vi "rsscope_core_global.vi"() -> ()   [LabVIEW 2014] (continued)
"Flags"=0, "Help"="DefiDefines, whether a search for any word length error (too few or too many bits per word) shall be activated or not.\n\nAvailable Repeated Capabilities:\nNone\n\nRemote-control command(s):\nSEARch:TRIGger:ETHernet:ERRor:LENGth"}, {"Level"=4, "Class Only"=TRUE, "Identifier"="", "Descriptive Name"="Results", "Data Type"=0, "Command"="", "Access"=0, "Range Table"="", "Read Callback"="", "Write Callback"="", "Supported Models"="", "Instrument Options"="", "Flags"=0, "Help"="Returns the search result of the specified word."}, {"Level"=5, "Class Only"=FALSE, "Identifier"="RSSCOPE_ATTR_SEARCH_ETHERNET_WORD_COUNT", "Descriptive Name"="Search Ethernet Word Count", "Data Type"=0, "Command"="SEAR:RES:ETH:WCO?", "Access"=0, "Range Table"="", "Read Callback"="rsscope_FormatSearchNameInt32_ReadCallback.vi", "Write Callback"="", "Supported Models"="", "Instrument Options"="K8", "Flags"=0, "Help"="Returns the number of decoded words.\n\nAvailable Repeated Capabilities:\nNone\n\nRemote-control command(s):\nSEARch:RESult:ETHernet:WCOunt?"}, {"Level"=3, "Class Only"=TRUE, "Identifier"="", "Descriptive Name"="USB", "Data Type"=0, "Command"="", "Access"=0, "Range Table"="", "Read Callback"="", "Write Callback"="", "Supported Models"="", "Instrument Options"="", "Flags"=0, "Help"="Configures USB search settings."}, {"Level"=4, "Class Only"=FALSE, "Identifier"="RSSCOPE_ATTR_SEARCH_USB_CRITERIA_START_OF_PACKET", "Descriptive Name"="Search USB Criteria Start Of Packet", "Data Type"=3, "Command"="SEAR:TRIG:USB:SSOP", "Access"=2, "Range Table"="", "Read Callback"="rsscope_FormatSearchNameBoolean_ReadCallback.vi", "Write Callback"="rsscope_FormatSearchNameBoolean_WriteCallback.vi", "Supported Models"="", "Instrument Options"="K60", "Flags"=0, "Help"="Defines, whether a start of packet (SOP) search shall be activated or not.\n\nAvailable Repeated Capabilities:\nNone\n\nRemote-control command(s):\nSEARch:TRIGger:USB:SSOP"}, {"Level"=4, "Class Only"=FALSE, "Identifier"="RSSCOPE_ATTR_SEARCH_USB_CRITERIA_TOKEN", "Descriptive Name"="Search USB Criteria Token", "Data Type"=3, "Command"="SEAR:TRIG:USB:STOK", "Access"=2, "Range Table"="", "Read Callback"="rsscope_FormatSearchNameBoolean_ReadCallback.vi", "Write Callback"="rsscope_FormatSearchNameBoolean_WriteCallback.vi", "Supported Models"="", "Instrument Options"="K60", "Flags"=0, "Help"="Defines, whether a search for any token packet shall be activated or not.\n\nAvailable Repeated Capabilities:\nNone\n\nRemote-control command(s):\nSEARch:TRIGger:USB:STOKen"}, {"Level"=4, "Class Only"=FALSE, "Identifier"="RSSCOPE_ATTR_SEARCH_USB_CRITERIA_DATA", "Descriptive Name"="Search USB Criteria Data", "Data Type"=3, "Command"="SEAR:TRIG:USB:SDAT", "Access"=2, "Range Table"="", "Read Callback"="rsscope_FormatSearchNameBoolean_ReadCallback.vi", "Write Callback"="rsscope_FormatSearchNameBoolean_WriteCallback.vi", "Supported Models"="", "Instrument Options"="K60", "Flags"=0, "Help"="Defines, whether the search for any data packet shall be activated or not.\n\nAvailable Repeated Capabilities:\nNone\n\nRemote-control command(s):\nSEARch:TRIGger:USB:SDATa"}, {"Level"=4, "Class Only"=FALSE, "Identifier"="RSSCOPE_ATTR_SEARCH_USB_CRITERIA_HANDSHAKE", "Descriptive Name"="Search USB Criteria Handshake", "Data Type"=3, "Command"="SEAR:TRIG:USB:SHAN", "Access"=2, "Range Table"="", "Read Callback"="rsscope_FormatSearchNameBoolean_ReadCallback.vi", "Write Callback"="rsscope_FormatSearchNameBoolean_WriteCallback.vi", "Supported Models"="", "Instrument Options"="K60", "Flags"=0, "Help"="Defines, whether the search for any handshake packet shall be activated or not.\n\nAvailable Repeated Capabilities:\nNone\n\nRemote-control command(s):\nSEARch:TRIGger:USB:SHANdshake"}, {"Level"=4, "Class Only"=FALSE, "Identifier"="RSSCOPE_ATTR_SEARCH_USB_CRITERIA_SPECIAL_PID", "Descriptive Name"="Search USB Criteria Special PID", "Data Type"=3, "Command"="SEAR:TRIG:USB:SSPE", "Access"=2, "Range Table"="", "Read Callback"="rsscope_FormatSearchNameBoolean_ReadCallback.vi", "Write Callback"="rsscope_FormatSearchNameBoolean_WriteCallback.vi", "Supported Models"="", "Instrument Options"="K60", "Flags"=0, "Help"="Defines, whether the search for any special PID packet shall be activated or not.\n\nAvailable Repeated Capabilities:\nNone\n\nRemote-control command(s):\nSEARch:TRIGger:USB:SSPE"}, {"Level"=4, "Class Only"=FALSE, "Identifier"="RSSCOPE_ATTR_SEARCH_USB_CRITERIA_ERROR", "Descriptive Name"="Search USB Criteria Error", "Data Type"=3, "Command"="SEAR:TRIG:USB:SERR", "Access"=2, "Range Table"="", "Read Callback"="rsscope_FormatSearchNameBoolean_ReadCallback.vi", "Write Callback"="rsscope_FormatSearchNameBoolean_WriteCallback.vi", "Supported Models"="", "Instrument Options"="K60", "Flags"=0, "Help"="Defines, whether the search for any error condition shall be activated or not.\n\nAvailable Repeated Capabilities:\nNone\n\nRemote-control command(s):\nSEARch:TRIGger:USB:SERRor"}, {"Level"=4, "Class Only"=FALSE, "Identifier"="RSSCOPE_ATTR_SEARCH_USB_TOKEN", "Descriptive Name"="Search USB Token", "Data Type"=0, "Command"="SEAR:TRIG:USB:TOK", "Access"=2, "Range Table"="rsscope_rngProtocolUSBSearchToken", "Read Callback"="rsscope_FormatSearchNameInt32_ReadCallback.vi", "Write Callback"="rsscope_FormatSearchNameInt32_WriteCallback.vi", "Supported Models"="", "Instrument Options"="K60", "Flags"=0, "Help"="Defines which token packet type is searched for: Out, In, Start Of Frame, Setup, or any token packet.\n\nAvailable Repeated Capabilities:\nNone\n\nRemote-control command(s):\nSEARch:TRIGger:USB:TOKen"}, {"Level"=4, "Class Only"=FALSE, "Identifier"="RSSCOPE_ATTR_SEARCH_USB_DATA_TYPE", "Descriptive Name"="Search USB Data Type", "Data Type"=0, "Command"="SEAR:TRIG:USB:DATA", "Access"=2, "Range Table"="rsscope_rngProtocolUSBSearchDataType", "Read Callback"="rsscope_FormatSearchNameInt32_ReadCallback.vi", "Write Callback"="rsscope_FormatSearchNameInt32_WriteCallback.vi", "Supported Models"="", "Instrument Options"="K60", "Flags"=0, "Help"="Defines, which data packet type is searched for: &apos;DATA0&apos;, &apos;DATA1&apos;, &apos;DATA2&apos;, or &apos;MDATA&apos;, as well as &apos;Any&apos; data packet.\n\nAvailable Repeated Capabilities:\nNone\n\nRemote-control command(s):\nSEARch:TRIGger:USB:DATA"}, {"Level"=4, "Class Only"=FALSE, "Identifier"="RSSCOPE_ATTR_SEARCH_USB_HANDSHAKE", "Descriptive Name"="Search USB Handshake", "Data Type"=0, "Command"="SEAR:TRIG:USB:HAND", "Access"=2, "Range Table"="rsscope_rngProtocolUSBTriggerHandshake", "Read Callback"="rsscope_FormatSearchNameInt32_ReadCallback.vi", "Write Callback"="rsscope_FormatSearchNameInt32_WriteCallback.vi", "Supported Models"="", "Instrument Options"="", "Flags"=0, "Help"="Defines, which handshake type is searched for.\n\nAvailable Repeated Capabilities:\nNone\n\nRemote-control command(s):\nSEARch:TRIGger:USB:HAND"}, {"Level"=4, "Class Only"=FALSE, "Identifier"="RSSCOPE_ATTR_SEARCH_USB_SPECIAL_PID", "Descriptive Name"="Search USB Special PID", "Data Type"=0, "Command"="SEAR:TRIG:USB:SPEC", "Access"=2, "Range Table"="rsscope_rngProtocolUSBSearchSpecialPID", "Read Callback"="rsscope_FormatSearchNameInt32_ReadCallback.vi", "Write Callback"="rsscope_FormatSearchNameInt32_WriteCallback.vi", "Supported Models"="", "Instrument Options"="K60", "Flags"=0, "Help"="Defines, which special PID packet type is searched for: &apos;PREamble&apos;, &apos;ERR&apos;, &apos;SPLit&apos;, &apos;PING&apos;, or &apos;Any&apos; special PID packet.\n\nAvailable Repeated Capabilities:\nNone\n\nRemote-control command(s):\nSEARch:TRIGger:USB:SPEC"}, {"Level"=4, "Class Only"=FALSE, "Identifier"="RSSCOPE_ATTR_SEARCH_USB_PID_ERROR_CHECK", "Descriptive Name"="Search USB PID Error Check", "Data Type"=3, "Command"="SEAR:TRIG:USB:WPID", "Access"=2, "Range Table"="", "Read Callback"="rsscope_FormatSearchNameBoolean_ReadCallback.vi", "Write Callback"="rsscope_FormatSearchNameBoolean_WriteCallback.vi", "Supported Models"="", "Instrument Options"="K60", "Flags"=0, "Help"="Defines, whether the packet ID error check shall be activated or not.\n\nAvailable Repeated Capabilities:\nNone\n\nRemote-control command(s):\nSEARch:TRIGger:USB:WPID"}, {"Level"=4, "Class Only"=TRUE, "Identifier"="", "Descriptive Name"="Error Condition", "Data Type"=0, "Command"="", "Access"=0, "Range Table"="", "Read Callback"="", "Write Callback"="", "Supported Models"="", "Instrument Options"="", "Flags"=0, "Help"="Configures error conditions to be searched."}, {"Level"=5, "Class Only"=FALSE, "Identifier"="RSSCOPE_ATTR_SEARCH_USB_ERROR_PID", "Descriptive Name"="Search USB Error PID", "Data Type"=3, "Command"="SEAR:TRIG:USB:PID", "Access"=2, "Range Table"="", "Read Callback"="rsscope_FormatSearchNameBoolean_ReadCallback.vi", "Write Callback"="rsscope_FormatSearchNameBoolean_WriteCallback.vi", "Supported Models"="", "Instrument Options"="K60", "Flags"=0, "Help"="Defines, whether a search for any PID error shall be activated or not.\n\nAvailable Repeated Capabilities:\nNone\n\nRemote-control command(s):\nSEARch:TRIGger:USB:PIDerror"}, {"Level"=5, "Class Only"=FALSE, "Identifier"="RSSCOPE_ATTR_SEARCH_USB_ERROR_CRC5", "Descriptive Name"="Search USB Error CRC5", "Data Type"=3, "Command"="SEAR:TRIG:USB:CRC5error", "Access"=2, "Range Table"="", "Read Callback"="rsscope_FormatSearchNameBoolean_ReadCallback.vi", "Write Callback"="rsscope_FormatSearchNameBoolean_WriteCallback.vi", "Supported Models"="", "Instrument Options"="K60", "Flags"=0, "Help"="Defines, whether a search for any CRC5 error shall be activated or not.\n\nAvailable Repeated Capabilities:\nNone\n\nRemote-control command(s):\nSEARch:TRIGger:USB:CRC5error"}, {"Level"=5, "Class Only"=FALSE, "Identifier"="RSSCOPE_ATTR_SEARCH_USB_ERROR_CRC16", "Descriptive Name"="Search USB Error CRC16", "Data Type"=3, "Command"="SEAR:TRIG:USB:CRC16error", "Access"=2, "Range Table"="", "Read Callback"="rsscope_FormatSearchNameBoolean_ReadCallback.vi", "Write Callback"="rsscope_FormatSearchNameBoolean_WriteCallback.vi", "Supported Models"="", "Instrument Options"="K60", "Flags"=0, "Help"="Defines, whether a search for any CRC16 error shall be activated or not.\n\nAvailable Repeated Capabilities:\nNone\n\nRemote-control command(s):\nSEARch:TRIGger:USB:CRC16error"}, {"Level"=5, "Class Only"=FALSE, "Identifier"="RSSCOPE_ATTR_SEARCH_USB_ERROR_BITSTUFF", "Descriptive Name"="Search USB Error Bitstuff", "Data Type"=3, "Command"="SEAR:TRIG:USB:BITS", "Access"=2, "Range Table"="", "Read Callback"="rsscope_FormatSearchNameBoolean_ReadCallback.vi", "Write Callback"="rsscope_FormatSearchNameBoolean_WriteCallback.vi", "Supported Models"="", "Instrument Options"="K60", "Flags"=0, "Help"="Defines, whether a search for any bitstuffing error shall be activated or not.\n\nAvailable Repeated Capabilities:\nNone\n\nRemote-control command(s):\nSEARch:TRIGger:USB:BITSterror"}, {"Level"=5, "Class Only"=FALSE, "Identifier"="RSSCOPE_ATTR_SEARCH_USB_ERROR_GLITCH", "Descriptive Name"="Search USB Error Glitch", "Data Type"=3, "Command"="SEAR:TRIG:USB:GLIT", "Access"=2, "Range Table"="", "Read Callback"="rsscope_FormatSearchNameBoolean_ReadCallback.vi", "Write Callback"="rsscope_FormatSearchNameBoolean_WriteCallback.vi", "Supported Models"="", "Instrument Options"="K60", "Flags"=0, "Help"="Defines, whether a search for any glitch error shall be activated or not.\n\nAvailable Repeated Capabilities:\nNone\n\nRemote-control command(s):\nSEARch:TRIGger:USB:GLITcherror"}, {"Level"=4, "Class Only"=TRUE, "Identifier"="", "Descriptive Name"="End Point Check", "Data Type"=0, "Command"="", "Access"=0, "Range Table"="", "Read Callback"="", "Write Callback"="", "Supported Models"="", "Instrument Options"="", "Flags"=0, "Help"="Defines, whether an endpoint check that meets specific conditions is executed or not."}, {"Level"=5, "Class Only"=FALSE, "Identifier"="RSSCOPE_ATTR_SEARCH_USB_END_POINT_CHECK", "Descriptive Name"="Search USB End Point Check", "Data Type"=3, "Command"="SEAR:TRIG:USB:WEND", "Access"=2, "Range Table"="", "Read Callback"="rsscope_FormatSearchNameBoolean_ReadCallback.vi", "Write Callback"="rsscope_FormatSearchNameBoolean_WriteCallback.vi", "Supported Models"="", "Instrument Options"="K60", "Flags"=0, "Help"="Defines, whether the endpoint check shall be activated or not.\n\nAvailable Repeated Capabilities:\nNone\n\nRemote-control command(s):\nSEARch:TRIGger:USB:WEND"}, {"Level"=5, "Class Only"=FALSE, "Identifier"="RSSCOPE_ATTR_SEARCH_USB_END_POINT_CHECK_CONDITION", "Descriptive Name"="Search USB End Point Check Condition", "Data Type"=0, "Command"="SEAR:TRIG:USB:ECON", "Access"=2, "Range Table"="rsscope_rngProtocolTriggerCondition", "Read Callback"="rsscope_FormatSearchNameInt32_ReadCallback.vi", "Write Callback"="rsscope_FormatSearchNameInt32_WriteCallback.vi", "Supported Models"="", "Instrument Options"="K60", "Flags"=0, "Help"="Sets the operator to set a specific endpoint or an endpoint range.\n\nAvailable Repeated Capabilities:\nNone\n\nRemote-control command(s):\nSEARch:TRIGger:USB:ECONdition"}, {"Level"=5, "Class Only"=FALSE, "Identifier"="RSSCOPE_ATTR_SEARCH_USB_END_POINT_CHECK_MIN", "Descriptive Name"="Search USB End Point Check Min", "Data Type"=2, "Command"="SEAR:TRIG:USB:EMIN", "Access"=1, "Range Table"="", "Read Callback"="", "Write Callback"="rsscope_FormatSearchNameString_WriteCallback.vi", "Supported Models"="", "Instrument Options"="K60", "Flags"=0, "Help"="Specifies the endpoint, or sets the start value of an endpoint range.\n\nAvailable Repeated Capabilities:\nNone\n\nRemote-control command(s):\nSEARch:TRIGger:USB:EMIN"}, {"Level"=5, "Class Only"=FALSE, "Identifier"="RSSCOPE_ATTR_SEARCH_USB_END_POINT_CHECK_MAX", "Descriptive Name"="Search USB End Point Check Max", "Data Type"=2, "Command"="SEAR:TRIG:USB:EMAX", "Access"=1, "Range Table"="", "Read Callback"="", "Write Callback"="rsscope_FormatSearchNameString_WriteCallback.vi", "Supported Models"="", "Instrument Options"="K60", "Flags"=0, "Help"="Sets the end value of an endpoint range if the corresponding condition is set to 'In range' and 'Out of range'.\n\nAvailable Repeated Capabilities:\nNone\n\nRemote-control command(s):\nSEARch:TRIGger:USB:EMAX"}, {"Level"=4, "Class Only"=TRUE, "Identifier"="", "Descriptive Name"="Address Check", "Data Type"=0, "Command"="", "Access"=0, "Range Table"="", "Read Callback"="", "Write Callback"="", "Supported Models"="", "Instrument Options"="", "Flags"=0, "Help"="Defines, whether an address check that meets specific conditions is executed or not."}, {"Level"=5, "Class Only"=FALSE, "Identifier"="RSSCOPE_ATTR_SEARCH_USB_ADDRESS_CHECK", "Descriptive Name"="Search USB Address Check", "Data Type"=3, "Command"="SEAR:TRIG:USB:WADD", "Access"=2, "Range Table"="", "Read Callback"="rsscope_FormatSearchNameBoolean_ReadCallback.vi", "Write Callback"="rsscope_FormatSearchNameBoolean_WriteCallback.vi", "Supported Models"="", "Instrument Options"="K60", "Flags"=0, "Help"="Defines, whether the address check shall be activated or not.\n\nAvailable Repeated Capabilities:\nNone\n\nRemote-control command(s):\nSEARch:TRIGger:USB:WADD"}, {"Level"=5, "Class Only"=FALSE, "Identifier"="RSSCOPE_ATTR_SEARCH_USB_ADDRESS_CHECK_CONDITION", "Descriptive Name"="Search USB Address Check Condition", "Data Type"=0, "Command"="SEAR:TRIG:USB:ACON", "Access"=2, "Range Table"="rsscope_rngProtocolTriggerCondition", "Read Callback"="rsscope_FormatSearchNameInt32_ReadCallback.vi", "Write Callback"="rsscope_FormatSearchNameInt32_WriteCallback.vi", "Supported Models"="", "Instrument Options"="K60", "Flags"=0, "Help"="Sets the operator to set a specific endpoint or an endpoint range.\n\nAvailable Repeated Capabilities:\nNone\n\nRemote-control command(s):\nSEARch:TRIGger:USB:ACONdition"}, {"Level"=5, "Class Only"=FALSE, "Identifier"="RSSCOPE_ATTR_SEARCH_USB_ADDRESS_CHECK_MIN", "Descriptive Name"="Search USB Address Check Min", "Data Type"=2, "Command"="SEAR:TRIG:USB:AMIN", "Access"=1, "Range Table"="", "Read Callback"="", "Write Callback"="rsscope_FormatSearchNameString_WriteCallback.vi", "Supported Models"="", "Instrument Options"="K60", "Flags"=0, "Help"="Specifies the address, or sets the start value of an address range.\n\nAvailable Repeated Capabilities:\nNone\n\nRemote-control command(s):\nSEARch:TRIGger:USB:AMIN"}, {"Level"=5, "Class Only"=FALSE, "Identifier"="RSSCOPE_ATTR_SEARCH_USB_ADDRESS_CHECK_MAX", "Descriptive Name"="Search USB Address Check Max", "Data Type"=2, "Command"="SEAR:TRIG:USB:AMAX", "Access"=1, "Range Table"="", "Read Callback"="", "Write Callback"="rsscope_FormatSearchNameString_WriteCallback.vi", "Supported Models"="", "Instrument Options"="K60", "Flags"=0, "Help"="Sets the end value of an address range if the corresponding condition is set to &apos;In range&apos; and &apos;Out of range&apos;.\n\nAvailable Repeated Capabilities:\nNone\n\nRemote-control command(s):\nSEARch:TRIGger:USB:AMAX"}, {"Level"=4, "Class Only"=TRUE, "Identifier"="", "Descriptive Name"="Payload Check", "Data Type"=0, "Command"="", "Access"=0, "Range Table"="", "Read Callback"="", "Write Callback"="", "Supported Models"="", "Instrument Options"="", "Flags"=0, "Help"="Defines, whether a payload check that meets specific conditions is executed or not."}, {"Level"=5, "Class Only"=FALSE, "Identifier"="RSSCOPE_ATTR_SEARCH_USB_PAYLOAD_CHECK", "Descriptive Name"="Search USB Payload Check", "Data Type"=3, "Command"="SEAR:TRIG:USB:WPAY", "Access"=2, "Range Table"="", "Read Callback"="rsscope_FormatSearchNameBoolean_ReadCallback.vi", "Write Callback"="rsscope_FormatSearchNameBoolean_WriteCallback.vi", "Supported Models"="", "Instrument Options"="K60", "Flags"=0, "Help"="Defines, whether the payload data check shall be activated or not.\n\nAvailable Repeated Capabilities:\nNone\n\nRemote-control command(s):\nSEARch:TRIGger:USB:WPAY"}, {"Level"=5, "Class Only"=FALSE, "Identifier"="RSSCOPE_ATTR_SEARCH_USB_PAYLOAD_CHECK_CONDITION", "Descriptive Name"="Search USB Payload Check Condition", "Data Type"=0, "Command"="SEAR:TRIG:USB:DPOP", "Access"=2, "Range Table"="rsscope_rngProtocolUSBPayloadCondition", "Read Callback"="rsscope_FormatSearchNameInt32_ReadCallback.vi", "Write Callback"="rsscope_FormatSearchNameInt32_WriteCallback.vi", "Supported Models"="", "Instrument Options"="K60", "Flags"=0, "Help"="Sets the operator to set a specific endpoint or an endpoint range.\n\nAvailable Repeated Capabilities:\nNone\n\nRemote-control command(s):\nSEARch:TRIGger:USB:DPOPerator"}, {"Level"=5, "Class Only"=FALSE, "Identifier"="RSSCOPE_ATTR_SEARCH_USB_PAYLOAD_CHECK_POSITION", "Descriptive Name"="Search USB Payload Check Position", "Data Type"=0, "Command"="SEAR:TRIG:USB:DPOS", "Access"=2, "Range Table"="rsscope_rngProtocolUSBPayloadPosition", "Read Callback"="rsscope_FormatSearchNameInt32_ReadCallback.vi", "Write Callback"="rsscope_FormatSearchNameInt32_WriteCallback.vi", "Supported Models"="", "Instrument Options"="K60", "Flags"=0, "Help"="Specifies the position within a payload data packet, in which a special data pattern is to be searched.\n\nAvailable Repeated Capabilities:\nNone\n\nRemote-control command(s):\nSEARch:TRIGger:USB:DPOSition"}, {"Level"=5, "Class Only"=FALSE, "Identifier"="RSSCOPE_ATTR_SEARCH_USB_PAYLOAD_CHECK_DATA_CONDITION", "Descriptive Name"="Search USB Payload Check Data Condition", "Data Type"=0, "Command"="SEAR:TRIG:USB:DCON", "Access"=2, "Range Table"="rsscope_rngNqEq", "Read Callback"="rsscope_FormatSearchNameInt32_ReadCallback.vi", "Write Callback"="rsscope_FormatSearchNameInt32_WriteCallback.vi", "Supported Models"="", "Instrument Options"="K60", "Flags"=0, "Help"="Sets the operator (equal or unequal) to set a specific payload data pattern.\n\nAvailable Repeated Capabilities:\nNone\n\nRemote-control command(s):\nSEARch:TRIGger:USB:DCONdition"}, {"Level"=5, "Class Only"=FALSE, "Identifier"="RSSCOPE_ATTR_SEARCH_USB_PAYLOAD_CHECK_PATTERN", "Descriptive Name"="Search USB Payload Check Pattern", "Data Type"=2, "Command"="SEAR:TRIG:USB:PATT", "Access"=1, "Range Table"="", "Read Callback"="", "Write Callback"="rsscope_FormatSearchNameString_WriteCallback.vi", "Supported Models"="", "Instrument Options"="K60", "Flags"=0, "Help"="Specifies the payload data pattern that is to be searched.\n\nAvailable Repeated Capabilities:\nNone\n\nRemote-control command(s):\nSEARch:TRIGger:USB:PATT"}, {"Level"=4, "Class Only"=TRUE, "Identifier"="", "Descriptive Name"="Frame Check", "Data Type"=0, "Command"="", "Access"=0, "Range Table"="", "Read Callback"="", "Write Callback"="", "Supported Models"="", "Instrument Options"="", "Flags"=0, "Help"="Defines, whether a frame number check that meets specific conditions is executed or not."}, {"Level"=5, "Class Only"=FALSE, "Identifier"="RSSCOPE_ATTR_SEARCH_USB_FRAME_CHECK", "Descriptive Name"="Search USB Frame Check", "Data Type"=3, "Command"="SEAR:TRIG:USB:WFRN", "Access"=2, "Range Table"="", "Read Callback"="rsscope_FormatSearchNameBoolean_ReadCallback.vi", "Write Callback"="rsscope_FormatSearchNameBoolean_WriteCallback.vi", "Supported Models"="", "Instrument Options"="K60", "Flags"=0, "Help"="Defines, whether the frame number check shall be activated or not.\n\nAvailable Repeated Capabilities:\nNone\n\nRemote-control command(s):\nSEARch:TRIGger:USB:WFRN"}, {"Level"=5, "Class Only"=FALSE, "Identifier"="RSSCOPE_ATTR_SEARCH_USB_FRAME_CHECK_CONDITION", "Descriptive Name"="Search USB Frame Check Condition", "Data Type"=0, "Command"="SEAR:TRIG:USB:FCON", "Access"=2, "Range Table"="rsscope_rngProtocolTriggerCondition", "Read Callback"="rsscope_FormatSearchNameInt32_ReadCallback.vi", "Write Callback"="rsscope_FormatSearchNameInt32_WriteCallback.vi", "Supported Models"="", "Instrument Options"="K60", "Flags"=0, "Help"="Sets the operator to set a specific frame number or a frame number range.\n\nAvailable Repeated Capabilities:\nNone\n\nRemote-control command(s):\nSEARch:TRIGger:USB:FCONdition"}, {"Level"=5, "Class Only"=FALSE, "Identifier"="RSSCOPE_ATTR_SEARCH_USB_FRAME_CHECK_MIN", "Descriptive Name"="Search USB Frame Check Min", "Data Type"=2, "Command"="SEAR:TRIG:USB:FMIN", "Access"=1, "Range Table"="", "Read Callback"="", "Write Callback"="rsscope_FormatSearchNameString_WriteCallback.vi", "Supported Models"="", "Instrument Options"="K60", "Flags"=0, "Help"="Specifies the frame number, or sets the start value of a frame number range.\n\nAvailable Repeated Capabilities:\nNone\n\nRemote-control command(s):\nSEARch:TRIGger:USB:FMIN"}, {"Level"=5, "Class Only"=FALSE, "Identifier"="RSSCOPE_ATTR_SEARCH_USB_FRAME_CHECK_MAX", "Descriptive Name"="Search USB Frame Check Max", "Data Type"=2, "Command"="SEAR:TRIG:USB:FMAX", "Access"=1, "Range Table"="", "Read Callback"="", "Write Callback"="rsscope_FormatSearchNameString_WriteCallback.vi", "Supported Models"="", "Instrument Options"="K60", "Flags"=0, "Help"="Sets the end value of a frame number range if the corresponding condition is set to &apos;In range&apos; and &apos;Out of range&apos;.\n\nAvailable Repeated Capabilities:\nNone\n\nRemote-control command(s):\nSEARch:TRIGger:USB:FMAX"}, {"Level"=4, "Class Only"=TRUE, "Identifier"="", "Descriptive Name"="SC Check", "Data Type"=0, "Command"="", "Access"=0, "Range Table"="", "Read Callback"="", "Write Callback"="", "Supported Models"="", "Instrument Options"="", "Flags"=0, "Help"="Defines, whether a Start / Complete SPLIT transaction check is executed or not."}, {"Level"=5, "Class Only"=FALSE, "Identifier"="RSSCOPE_ATTR_SEARCH_USB_SC_CHECK", "Descriptive Name"="Search USB SC Check", "Data Type"=3, "Command"="SEAR:TRIG:USB:WSTC", "Access"=2, "Range Table"="", "Read Callback"="rsscope_FormatSearchNameBoolean_ReadCallback.vi", "Write Callback"="rsscope_FormatSearchNameBoolean_WriteCallback.vi", "Supported Models"="", "Instrument Options"="K60", "Flags"=0, "Help"="Defines, whether the frame number check shall be activated or not.\n\nAvailable Repeated Capabilities:\nNone\n\nRemote-control command(s):\nSEARch:TRIGger:USB:WSTC"}, {"Level"=5, "Class Only"=FALSE, "Identifier"="RSSCOPE_ATTR_SEARCH_USB_SC_CHECK_START_COMPLETE", "Descriptive Name"="Search USB SC Check Start Complete", "Data Type"=0, "Command"="SEAR:TRIG:USB:STCO", "Access"=2, "Range Table"="rsscope_rngProtocolUSBSCCheckStartComplete", "Read Callback"="rsscope_FormatSearchNameInt32_ReadCallback.vi", "Write Callback"="rsscope_FormatSearchNameInt32_WriteCallback.vi", "Supported Models"="", "Instrument Options"="K60", "Flags"=0, "Help"="Sets the trigger to a specific start-split or complete-split transaction endpoint.\n\nAvailable Repeated Capabilities:\nNone\n\nRemote-control command(s):\nSEARch:TRIGger:USB:STCO"}, {"Level"=4, "Class Only"=TRUE, "Identifier"="", "Descriptive Name"="Port Check", "Data Type"=0, "Command"="", "Access"=0, "Range Table"="", "Read Callback"="", "Write Callback"="", "Supported Models"="", "Instrument Options"="", "Flags"=0, "Help"="Defines, whether a frame number check that meets specific conditions is executed or not."}, {"Level"=5, "Class Only"=FALSE, "Identifier"="RSSCOPE_ATTR_SEARCH_USB_PORT_CHECK", "Descriptive Name"="Search USB Port Check", "Data Type"=3, "Command"="SEAR:TRIG:USB:WPOR", "Access"=2, "Range Table"="", "Read Callback"="rsscope_FormatSearchNameBoolean_ReadCallback.vi", "Write Callback"="rsscope_FormatSearchNameBoolean_WriteCallback.vi", "Supported Models"="", "Instrument Options"="K60", "Flags"=0, "Help"="Defines, whether the port check shall be activated or not.\n\nAvailable Repeated Capabilities:\nNone\n\nRemote-control command(s):\nSEARch:TRIGger:USB:WPOR"}, {"Level"=5, "Class Only"=FALSE, "Identifier"="RSSCOPE_ATTR_SEARCH_USB_PORT_CHECK_CONDITION", "Descriptive Name"="Search USB Port Check Condition", "Data Type"=0, "Command"="SEAR:TRIG:USB:PCON", "Access"=2, "Range Table"="rsscope_rngProtocolTriggerCondition", "Read Callback"="rsscope_FormatSearchNameInt32_ReadCallback.vi", "Write Callback"="rsscope_FormatSearchNameInt32_WriteCallback.vi", "Supported Models"="", "Instrument Options"="K60", "Flags"=0, "Help"="Sets the operator to set a specific port number or a port number range.\n\nAvailable Repeated Capabilities:\nNone\n\nRemote-control command(s):\nSEARch:TRIGger:USB:PCONdition"}, {"Level"=5, "Class Only"=FALSE, "Identifier"="RSSCOPE_ATTR_SEARCH_USB_PORT_CHECK_MIN", "Descriptive Name"="Search USB Port Check Min", "Data Type"=2, "Command"="SEAR:TRIG:USB:PMIN", "Access"=1, "Range Table"="", "Read Callback"="", "Write Callback"="rsscope_FormatSearchNameString_WriteCallback.vi", "Supported Models"="", "Instrument Options"="K60", "Flags"=0, "Help"="Specifies the port number, or sets the start value of a port number range.\n\nAvailable Repeated Capabilities:\nNone\n\nRemote-control command(s):\nSEARch:TRIGger:USB:PMIN"}, {"Level"=5, "Class Only"=FALSE, "Identifier"="RSSCOPE_ATTR_SEARCH_USB_PORT_CHECK_MAX", "Descriptive Name"="Search USB Port Check Max", "Data Type"=2, "Command"="SEAR:TRIG:USB:PMAX", "Access"=1, "Range Table"="", "Read Callback"="", "Write Callback"="rsscope_FormatSearchNameString_WriteCallback.vi", "Supported Models"="", "Instrument Options"="K60", "Flags"=0, "Help"="Sets the end value of a port number range if the corresponding condition is set to 'In range' and 'Out of range'.\n\nAvailable Repeated Capabilities:\nNone\n\nRemote-control command(s):\nSEARch:TRIGger:USB:PMAX"}, {"Level"=4, "Class Only"=TRUE, "Identifier"="", "Descriptive Name"="SEU Check", "Data Type"=0, "Command"="", "Access"=0, "Range Table"="", "Read Callback"="", "Write Callback"="", "Supported Models"="", "Instrument Options"="", "Flags"=0, "Help"="Defines, whether an SEU check that meets specific conditions is executed or not. S and E represent the Start and End of a start-split transaction, U represents the reserved/Unused bit of a complete-split transaction. Permissible binary SEU values are 00, 01, 10, and 11."}, {"Level"=5, "Class Only"=FALSE, "Identifier"="RSSCOPE_ATTR_SEARCH_USB_SEU_CHECK", "Descriptive Name"="Search USB SEU Check", "Data Type"=3, "Command"="SEAR:TRIG:USB:WSEU", "Access"=2, "Range Table"="", "Read Callback"="rsscope_FormatSearchNameBoolean_ReadCallback.vi", "Write Callback"="rsscope_FormatSearchNameBoolean_WriteCallback.vi", "Supported Models"="", "Instrument Options"="K60", "Flags"=0, "Help"="Defines, whether the SEU check shall be activated or not.\n\nAvailable Repeated Capabilities:\nNone\n\nRemote-control command(s):\nSEARch:TRIGger:USB:WSEU"}, {"Level"=5, "Class Only"=FALSE, "Identifier"="RSSCOPE_ATTR_SEARCH_USB_SEU_CHECK_CONDITION", "Descriptive Name"="Search USB SEU Check Condition", "Data Type"=0, "Command"="SEAR:TRIG:USB:SCON", "Access"=2, "Range Table"="rsscope_rngProtocolTriggerCondition", "Read Callback"="rsscope_FormatSearchNameInt32_ReadCallback.vi", "Write Callback"="rsscope_FormatSearchNameInt32_WriteCallback.vi", "Supported Models"="", "Instrument Options"="K60", "Flags"=0, "Help"="Sets the operator to set a specific SEU or an SEU range.\n\nAvailable Repeated Capabilities:\nNone\n\nRemote-control command(s):\nSEARch:TRIGger:USB:SCONdition"}, {"Level"=5, "Class Only"=FALSE, "Identifier"="RSSCOPE_ATTR_SEARCH_USB_SEU_CHECK_MIN", "Descriptive Name"="Search USB SEU Check Min", "Data Type"=2, "Command"="SEAR:TRIG:USB:SMIN", "Access"=1, "Range Table"="", "Read Callback"="", "Write Callback"="rsscope_FormatSearchNameString_WriteCallback.vi", "Supported Models"="", "Instrument Options"="K60", "Flags"=0, "Help"="Specifies the SEU, or sets the start value of an SEU range.\n\nAvailable Repeated Capabilities:\nNone\n\nRemote-control command(s):\nSEARch:TRIGger:USB:SMIN"}, {"Level"=5, "Class Only"=FALSE, "Identifier"="RSSCOPE_ATTR_SEARCH_USB_SEU_CHECK_MAX", "Descriptive Name"="Search USB SEU Check Max", "Data Type"=2, "Command"="SEAR:TRIG:USB:SMAX", "Access"=1, "Range Table"="", "Read Callback"="", "Write Callback"="rsscope_FormatSearchNameString_WriteCallback.vi", "Supported Models"="", "Instrument Options"="K60", "Flags"=0, "Help"="Sets the end value of an SEU range if the corresponding condition is set to &apos;In range&apos; and &apos;Out of range&apos;.\n\nAvailable Repeated Capabilities:\nNone\n\nRemote-control command(s):\nSEARch:TRIGger:USB:SMAX"}, {"Level"=4, "Class Only"=TRUE, "Identifier"="", "Descriptive Name"="ET Check", "Data Type"=0, "Command"="", "Access"=0, "Range Table"="", "Read Callback"="", "Write Callback"="", "Supported Models"="", "Instrument Options"="", "Flags"=0, "Help"="Defines, whether an Endpoint Type (ET) check that meets specific conditions is executed or not."}, {"Level"=5, "Class Only"=FALSE, "Identifier"="RSSCOPE_ATTR_SEARCH_USB_ET_CHECK", "Descriptive Name"="Search USB ET Check", "Data Type"=3, "Command"="SEAR:TRIG:USB:WETC", "Access"=2, "Range Table"="", "Read Callback"="rsscope_FormatSearchNameBoolean_ReadCallback.vi", "Write Callback"="rsscope_FormatSearchNameBoolean_WriteCallback.vi", "Supported Models"="", "Instrument Options"="K60", "Flags"=0, "Help"="Defines, whether the Endpoint Type (ET) check shall be activated or not.\n\nAvailable Repeated Capabilities:\nNone\n\nRemote-control command(s):\nSEARch:TRIGger:USB:WETCheck"}, {"Level"=5, "Class Only"=FALSE, "Identifier"="RSSCOPE_ATTR_SEARCH_USB_ET_CHECK_CONDITION", "Descriptive Name"="Search USB ET Check Condition", "Data Type"=0, "Command"="SEAR:TRIG:USB:TCON", "Access"=2, "Range Table"="rsscope_rngProtocolTriggerCondition", "Read Callback"="rsscope_FormatSearchNameInt32_ReadCallback.vi", "Write Callback"="rsscope_FormatSearchNameInt32_WriteCallback.vi", "Supported Models"="", "Instrument Options"="K60", "Flags"=0, "Help"="Sets the operator to set a specific endpoint type (ET) or an ET range.\n\nAvailable Repeated Capabilities:\nNone\n\nRemote-control command(s):\nSEARch:TRIGger:USB:TCONdition"}, {"Level"=5, "Class Only"=FALSE, "Identifier"="RSSCOPE_ATTR_SEARCH_USB_ET_CHECK_MIN", "Descriptive Name"="Search USB ET Check Min", "Data Type"=2, "Command"="SEAR:TRIG:USB:TMIN", "Access"=1, "Range Table"="", "Read Callback"="", "Write Callback"="rsscope_FormatSearchNameString_WriteCallback.vi", "Supported Models"="", "Instrument Options"="K60", "Flags"=0, "Help"="Specifies the endpoint type, or sets the start value of an endpoint type range.\n\nAvailable Repeated Capabilities:\nNone\n\nRemote-control command(s):\nSEARch:TRIGger:USB:TMIN"}, {"Level"=5, "Class Only"=FALSE, "Identifier"="RSSCOPE_ATTR_SEARCH_USB_ET_CHECK_MAX", "Descriptive Name"="Search USB ET Check Max", "Data Type"=2, "Command"="SEAR:TRIG:USB:TMAX", "Access"=1, "Range Table"="", "Read Callback"="", "Write Callback"="rsscope_FormatSearchNameString_WriteCallback.vi", "Supported Models"="", "Instrument Options"="K60", "Flags"=0, "Help"="Sets the end value of an endpoint type range if the corresponding condition is set to &apos;In range&apos; and &apos;Out of range&apos;.\n\nAvailable Repeated Capabilities:\nNone\n\nRemote-control command(s):\nSEARch:TRIGger:USB:TMAX"}, {"Level"=4, "Class Only"=TRUE, "Identifier"="", "Descriptive Name"="Results", "Data Type"=0, "Command"="", "Access"=0, "Range Table"="", "Read Callback"="", "Write Callback"="", "Supported Models"="", "Instrument Options"="", "Flags"=0, "Help"="Returns the search result of the specified packet."}, {"Level"=5, "Class Only"=FALSE, "Identifier"="RSSCOPE_ATTR_SEARCH_USB_PACKET_COUNT", "Descriptive Name"="Search USB Packet Count", "Data Type"=0, "Command"="SEAR:RES:USB:PCO?", "Access"=0, "Range Table"="", "Read Callback"="rsscope_FormatSearchNameInt32_ReadCallback.vi", "Write Callback"="", "Supported Models"="", "Instrument Options"="K60", "Flags"=0, "Help"="Returns the packet count for the selected serial bus, i.e. the number of packets in the present acquisition.\n\nAvailable Repeated Capabilities:\nNone\n\nRemote-control command(s):\nSEARch:RESult:USB:PCOunt?"}, {"Level"=3, "Class Only"=TRUE, "Identifier"="", "Descriptive Name"="USB 31 Generation 1", "Data Type"=0, "Command"="", "Access"=0, "Range Table"="", "Read Callback"="", "Write Callback"="", "Supported Models"="", "Instrument Options"="", "Flags"=0, "Help"="Configures USB 3.1 Generation 1 search."}, {"Level"=4, "Class Only"=TRUE, "Identifier"="", "Descriptive Name"="Results", "Data Type"=0, "Command"="", "Access"=0, "Range Table"="", "Read Callback"="", "Write Callback"="", "Supported Models"="", "Instrument Options"="", "Flags"=0, "Help"="Searches the USB31 Generation1 decoding results."}, {"Level"=5, "Class Only"=FALSE, "Identifier"="RSSCOPE_ATTR_SEARCH_USB31_GEN1_FRAME_COUNT", "Descriptive Name"="Search USB31 Gen1 Frame Count", "Data Type"=0, "Command"="SEAR:RES:USBT:FCO?", "Access"=0, "Range Table"="", "Read Callback"="rsscope_FormatSearchNameInt32_ReadCallback.vi", "Write Callback"="", "Supported Models"="", "Instrument Options"="K61", "Flags"=0, "Help"="Returns the number of frames in the acquisition.\n\nAvailable Repeated Capabilities:\nNone\n\nRemote-control command(s):\nSEARch:RESult:USBThree:FCOunt?"}, {"Level"=3, "Class Only"=TRUE, "Identifier"="", "Descriptive Name"="USB PD", "Data Type"=0, "Command"="", "Access"=0, "Range Table"="", "Read Callback"="", "Write Callback"="", "Supported Models"="", "Instrument Options"="", "Flags"=0, "Help"="Configures USB PD  search."}, {"Level"=4, "Class Only"=FALSE, "Identifier"="RSSCOPE_ATTR_USB_PD_SEARCH_TYPE", "Descriptive Name"="USB PD Search Type", "Data Type"=0, "Command"="SEAR:TRIG:USBP:TYPE", "Access"=2, "Range Table"="RsScope_rngUSBPDTriggerType", "Read Callback"="rsscope_FormatSearchNameInt32_ReadCallback.vi", "Write Callback"="rsscope_FormatSearchNameInt32_WriteCallback.vi", "Supported Models"="", "Instrument Options"="K63", "Flags"=0, "Help"="Selects the trigger type.\n\nAvailable Repeated Capabilities:\nNone\n\nRemote-control command(s):\nSEARch:TRIGger:USBPd:TYPE"}, {"Level"=4, "Class Only"=FALSE, "Identifier"="RSSCOPE_ATTR_USB_PD_SEARCH_PACKET_TYPE", "Descriptive Name"="USB PD Search Packet Type", "Data Type"=0, "Command"="SEAR:TRIG:USBP:FRAM:SEL", "Access"=2, "Range Table"="RsScope_rngUSBPDPacketType", "Read Callback"="rsscope_empty_ReadCallback.vi", "Write Callback"="rsscope_FormatSearchNameInt32_WriteCallback.vi", "Supported Models"="", "Instrument Options"="K63", "Flags"=0, "Help"="Selects the frame to be triggered on, if the frame does not have any fields, e.g. a test frame.\n\nAvailable Repeated Capabilities:\nNone\n\nRemote-control command(s):\nSEARch:TRIGger:USBPd:FRAMe:SELect"}, {"Level"=4, "Class Only"=FALSE, "Identifier"="RSSCOPE_ATTR_USB_PD_SEARCH_NUMBER_OF_FRAMES", "Descriptive Name"="USB PD Search Number Of Frames", "Data Type"=0, "Command"="SEAR:RES:USBP:FCO?", "Access"=0, "Range Table"="", "Read Callback"="rsscope_FormatSearchNameInt32_ReadCallback.vi", "Write Callback"="", "Supported Models"="", "Instrument Options"="", "Flags"=0, "Help"="Returns the number of decoded frames in the search result.\n\nAvailable Repeated Capabilities:\nNone\n\nRemote-control command(s):\nSEARch:RESult:USBPd:FCOunt?"}, {"Level"=4, "Class Only"=TRUE, "Identifier"="", "Descriptive Name"="Data", "Data Type"=0, "Command"="", "Access"=0, "Range Table"="", "Read Callback"="", "Write Callback"="", "Supported Models"="", "Instrument Options"="", "Flags"=0, "Help"="Defines for the selected field, how a data check is executed."}, {"Level"=5, "Class Only"=FALSE, "Identifier"="RSSCOPE_ATTR_USB_PD_SEARCH_DATA_CONDITION", "Descriptive Name"="USB PD Search Data Condition", "Data Type"=0, "Command"="SEAR:TRIG:USBP:FRAM:FIEL{FieldNumber}:DOP", "Access"=2, "Range Table"="rsscope_rngProtocolTriggerCondition", "Read Callback"="rsscope_FormatUSBPDPacketTypeInt32_ReadCallback.vi", "Write Callback"="rsscope_FormatUSBPDPacketTypeInt32_WriteCallback.vi", "Supported Models"="", "Instrument Options"="K63", "Flags"=0, "Help"="Sets the condition for the data pattern. You can define no value, an exact value or a value range.\n\nAvailable Repeated Capabilities:\nFieldNumber: Field1, Field2, Field3, Field4, Field5, Field6, Field7, Field8, Field9, Field10, Field11, Field12, Field13, Field14, Field15, Field16, Field17, Field18, Field19, Field20\r\n\nRemote-control command(s):\nSEARch:TRIGger:USBPd:FRAMe:FIELd<m>:DOPerator"}, {"Level"=5, "Class Only"=FALSE, "Identifier"="RSSCOPE_ATTR_USB_PD_SEARCH_DATA_MIN", "Descriptive Name"="USB PD Search Data Min", "Data Type"=2, "Command"="SEAR:TRIG:USBP:FRAM:FIEL{FieldNumber}:DMIN", "Access"=2, "Range Table"="", "Read Callback"="rsscope_FormatUSBPDPacketTypeString_ReadCallback.vi", "Write Callback"="rsscope_FormatUSBPDPacketTypeString_WriteCallback.vi", "Supported Models"="", "Instrument Options"="K63", "Flags"=0, "Help"="Specifies a data bit pattern, or sets the start value of a pattern range.\n\nValid Values:\nBinary pattern string consisting of 1; 0; or X (any bit).\n\nAvailable Repeated Capabilities:\nFieldNumber: Field1, Field2, Field3, Field4, Field5, Field6, Field7, Field8, Field9, Field10, Field11, Field12, Field13, Field14, Field15, Field16, Field17, Field18, Field19, Field20\r\n\nRemote-control command(s):\nSEARch:TRIGger:USBPd:FRAMe:FIELd<m>:DMIN"}, {"Level"=5, "Class Only"=FALSE, "Identifier"="RSSCOPE_ATTR_USB_PD_SEARCH_DATA_MAX", "Descriptive Name"="USB PD Search Data Max", "Data Type"=2, "Command"="SEAR:TRIG:USBP:FRAM:FIEL{FieldNumber}:DMAX", "Access"=2, "Range Table"="", "Read Callback"="rsscope_FormatUSBPDPacketTypeString_ReadCallback.vi", "Write Callback"="rsscope_FormatUSBPDPacketTypeString_WriteCallback.vi", "Supported Models"="", "Instrument Options"="K63", "Flags"=0, "Help"="Sets the end value of a data type range for condition In Range or Out of Range. \n\nValid Values:\nBinary pattern string consisting of 1; 0; or X (any bit).\n\nAvailable Repeated Capabilities:\nFieldNumber: Field1, Field2, Field3, Field4, Field5, Field6, Field7, Field8, Field9, Field10, Field11, Field12, Field13, Field14, Field15, Field16, Field17, Field18, Field19, Field20\r\n\nRemote-control command(s):\nSEARch:TRIGger:USBPd:FRAMe:FIELd<m>:DMAX"}, {"Level"=4, "Class Only"=TRUE, "Identifier"="", "Descriptive Name"="Index", "Data Type"=0, "Command"="", "Access"=0, "Range Table"="", "Read Callback"="", "Write Callback"="", "Supported Models"="", "Instrument 
